vi "Close_loop_Position_Control_of_Tip.vi"() -> ()   [LabVIEW 2019]
uses:
  <vilib>/FPGAPlugInAG/sbRIO-9629/niLvFpga_Open_sbRIO-9629.vi
  <vilib>/rvi/interface/common/dynamic/niFpgaDynamicAddResources.vi
  <vilib>/imath/engines/lvmath2/RunTimeEngine/Managers/WorkSpace/UID Generator.vi
  <vilib>/imath/engines/lvmath2/RunTimeEngine/IndexRead/NIMS V(S).vi
  <instcachedir>/0/NIMS V(S)_0488751826AF41519A22953C041130DC.lvgen/NIMS V(S)_0488751826AF41519A22953C041130DC_000.vi
  <vilib>/imath/engines/lvmath2/RunTimeEngine/BuiltInFunctions/atan2/NIMS_atan2.vi
  <instcachedir>/0/NIMS_atan2_A91AA4A7D42247EDBE8F76DB99AF04A4.lvgen/NIMS_atan2_A91AA4A7D42247EDBE8F76DB99AF04A4_000.vi
  <vilib>/imath/engines/lvmath2/RunTimeEngine/RunTimeType/NIMS_RunTimeType_From StrictType (excl LVString).vi
  <instcachedir>/0/NIMS_RunTimeType_From StrictType (excl LVString)_D8AFBA86A94845AAA577C895450664BD.lvgen/NIMS_RunTimeType_From StrictType (excl LVString)_D8AFBA86A94845AAA577C895450664BD_000.vi
  <vilib>/imath/engines/lvmath2/RunTimeEngine/ErrorHandling/NIMS_Create Error From Enums.vi
  <vilib>/imath/engines/lvmath2/RunTimeEngine/LocalVariableDefStatement/MC_LocalVariableDefStatement_Display.vi
  <vilib>/imath/engines/lvmath2/RunTimeEngine/BuiltInFunctions/atan/NIMS_atan(C).vi
  <instcachedir>/0/NIMS_atan(C)_0A85D365582D4E8AB3874BC9125E138E.lvgen/NIMS_atan(C)_0A85D365582D4E8AB3874BC9125E138E_001.vi
  <vilib>/imath/engines/lvmath2/RunTimeEngine/BuiltInFunctions/cross/NIMS_cross(GV,GV).vi
  <instcachedir>/0/NIMS_cross(GV,GV)_6F1F1C643EFF41C8A983D972A94A5A15.lvgen/NIMS_cross(GV,GV)_6F1F1C643EFF41C8A983D972A94A5A15_000.vi
  <vilib>/imath/engines/lvmath2/RunTimeEngine/BuiltInFunctions/norm/NIMS_norm(GV,DBL).vi
  <instcachedir>/0/NIMS_norm(GV,DBL)_4A8B6F23BC0A47549B8AB805006257D9.lvgen/NIMS_norm(GV,DBL)_4A8B6F23BC0A47549B8AB805006257D9_000.vi
  <vilib>/imath/engines/lvmath2/RunTimeEngine/ArithmeticOperatorToken/NIMS_ArithmeticOperator_multmx-internal.vi
  <instcachedir>/0/NIMS_ArithmeticOperator_multmx-internal_9E91BA3A2DCB4083AAD724A04442A6F7.lvgen/NIMS_ArithmeticOperator_multmx-internal_9E91BA3A2DCB4083AAD724A04442A6F7_004.vi
  <vilib>/imath/engines/lvmath2/RunTimeEngine/BuiltInFunctions/cos/NIMS_cos(C).vi
  <instcachedir>/0/NIMS_cos(C)_BED070B05FDB4939A63CB05E18805866.lvgen/NIMS_cos(C)_BED070B05FDB4939A63CB05E18805866_001.vi
  <vilib>/imath/engines/lvmath2/RunTimeEngine/BuiltInFunctions/sin/NIMS_sin(C).vi
  <instcachedir>/0/NIMS_sin(C)_6504C6AC704B4661870B0E93397B11C4.lvgen/NIMS_sin(C)_6504C6AC704B4661870B0E93397B11C4_001.vi
  <vilib>/imathl/engines/lvmath/Functions/Error Handling/Create Error.vi
  <vilib>/imath/engines/lvmath2/RunTimeEngine/ArithmeticOperatorToken/NIMS_ArithmeticOperator_multmx(M,CV)-internal.vi
  <instcachedir>/0/NIMS_ArithmeticOperator_multmx(M,CV)-internal_2C55777844884EEDB828A940D397C7D0.lvgen/NIMS_ArithmeticOperator_multmx(M,CV)-internal_2C55777844884EEDB828A940D397C7D0_002.vi
  <instcachedir>/0/NIMS_norm(GV,DBL)_4A8B6F23BC0A47549B8AB805006257D9.lvgen/NIMS_norm(GV,DBL)_4A8B6F23BC0A47549B8AB805006257D9_001.vi
  <vilib>/imath/engines/lvmath2/RunTimeEngine/Managers/SymbolTable/Clear UID.vi
  <vilib>/imath/engines/lvmath2/RunTimeEngine/NodeEndStatement/NIMS_NodeEndStatement_Output.vi
  <instcachedir>/0/NIMS_NodeEndStatement_Output_53EC0D466D134D7ABD903AC30B43404B.lvgen/NIMS_NodeEndStatement_Output_53EC0D466D134D7ABD903AC30B43404B_001.vi
  <vilib>/imath/engines/lvmath2/RunTimeEngine/ErrorHandling/NIMS_Finalize Error.vi
  <vilib>/Utility/error.llb/Error Cluster From Error Code.vi
  <vilib>/rvi/errors/niLvFpgaAdjustHostInterfaceError.vi
  <vilib>/FPGAPlugInAG/Dynamic/niLvFpga_Close_Dynamic.vi
  <vilib>/rvi/interface/nirviOpenFPGA/nirviOpenFPGA.xnode
  FPGA Bitfiles/fcmsinglesection_FPGATarget_CloseLoopMotorTu_eGt+d+EV+VE.lvbitx
  Close_Loop_Motor_Tune.vi
  <vilib>/rvi/interface/nirviReadWriteControl/nirviReadWriteControl.xnode
  <vilib>/rvi/interface/nirviCloseFPGA/nirviCloseFPGA.xnode
  NiFpgaLv.dll
  <vilib>/rvi/interface/Simulation/niFpgaSimulationCallBeginRW.vi
  <vilib>/imath/engines/lvmath2/RunTimeEngine/Managers/SymbolTable/NIMS_WorkSpace.lvlib
panel:
  in  "Kp":dbl[](array[numeric])
  in  "Motor3_KP":sgl
  in  "Motor2_KP":sgl
  in  "Motor1_KP":sgl
  in  "Position Reset 2_e":bool
  out "Theta 3 (error)":dbl
  out "Theta 2 (error)":dbl
  out "Theta 1 (error)":dbl
  out "alpha (error)":dbl
  out "L_v (error)":dbl
  out "Error Indicator":bool
  out "Error":dbl[](array[numeric])
  out "error out 2":errorcluster
  out "Y Position(mm) marker 25":dbl
  out "X Position(mm) marker 25":dbl
  out "Z Position(mm) marker 25":dbl
  out "Actual Tip Coordinates(m)":dbl[](array[numeric])
  out "LED ID 2":i32
  out "FRAME 2":string
  out "data out 2":string
  in  "Desired Tip position (m)":dbl[](array[numeric])
  out "L1 (m)":dbl
  out "L2 (m)":dbl
  out "L3 (m)":dbl
  out "Theta 1":dbl
  out "Theta 2":dbl
  out "Theta 3":dbl
  in  "Position Reset":bool
  out "output variable":dbl
  out "output variable 2":dbl
  out "output variable 3":dbl
  out "alpha":dbl
  out "L_v":dbl
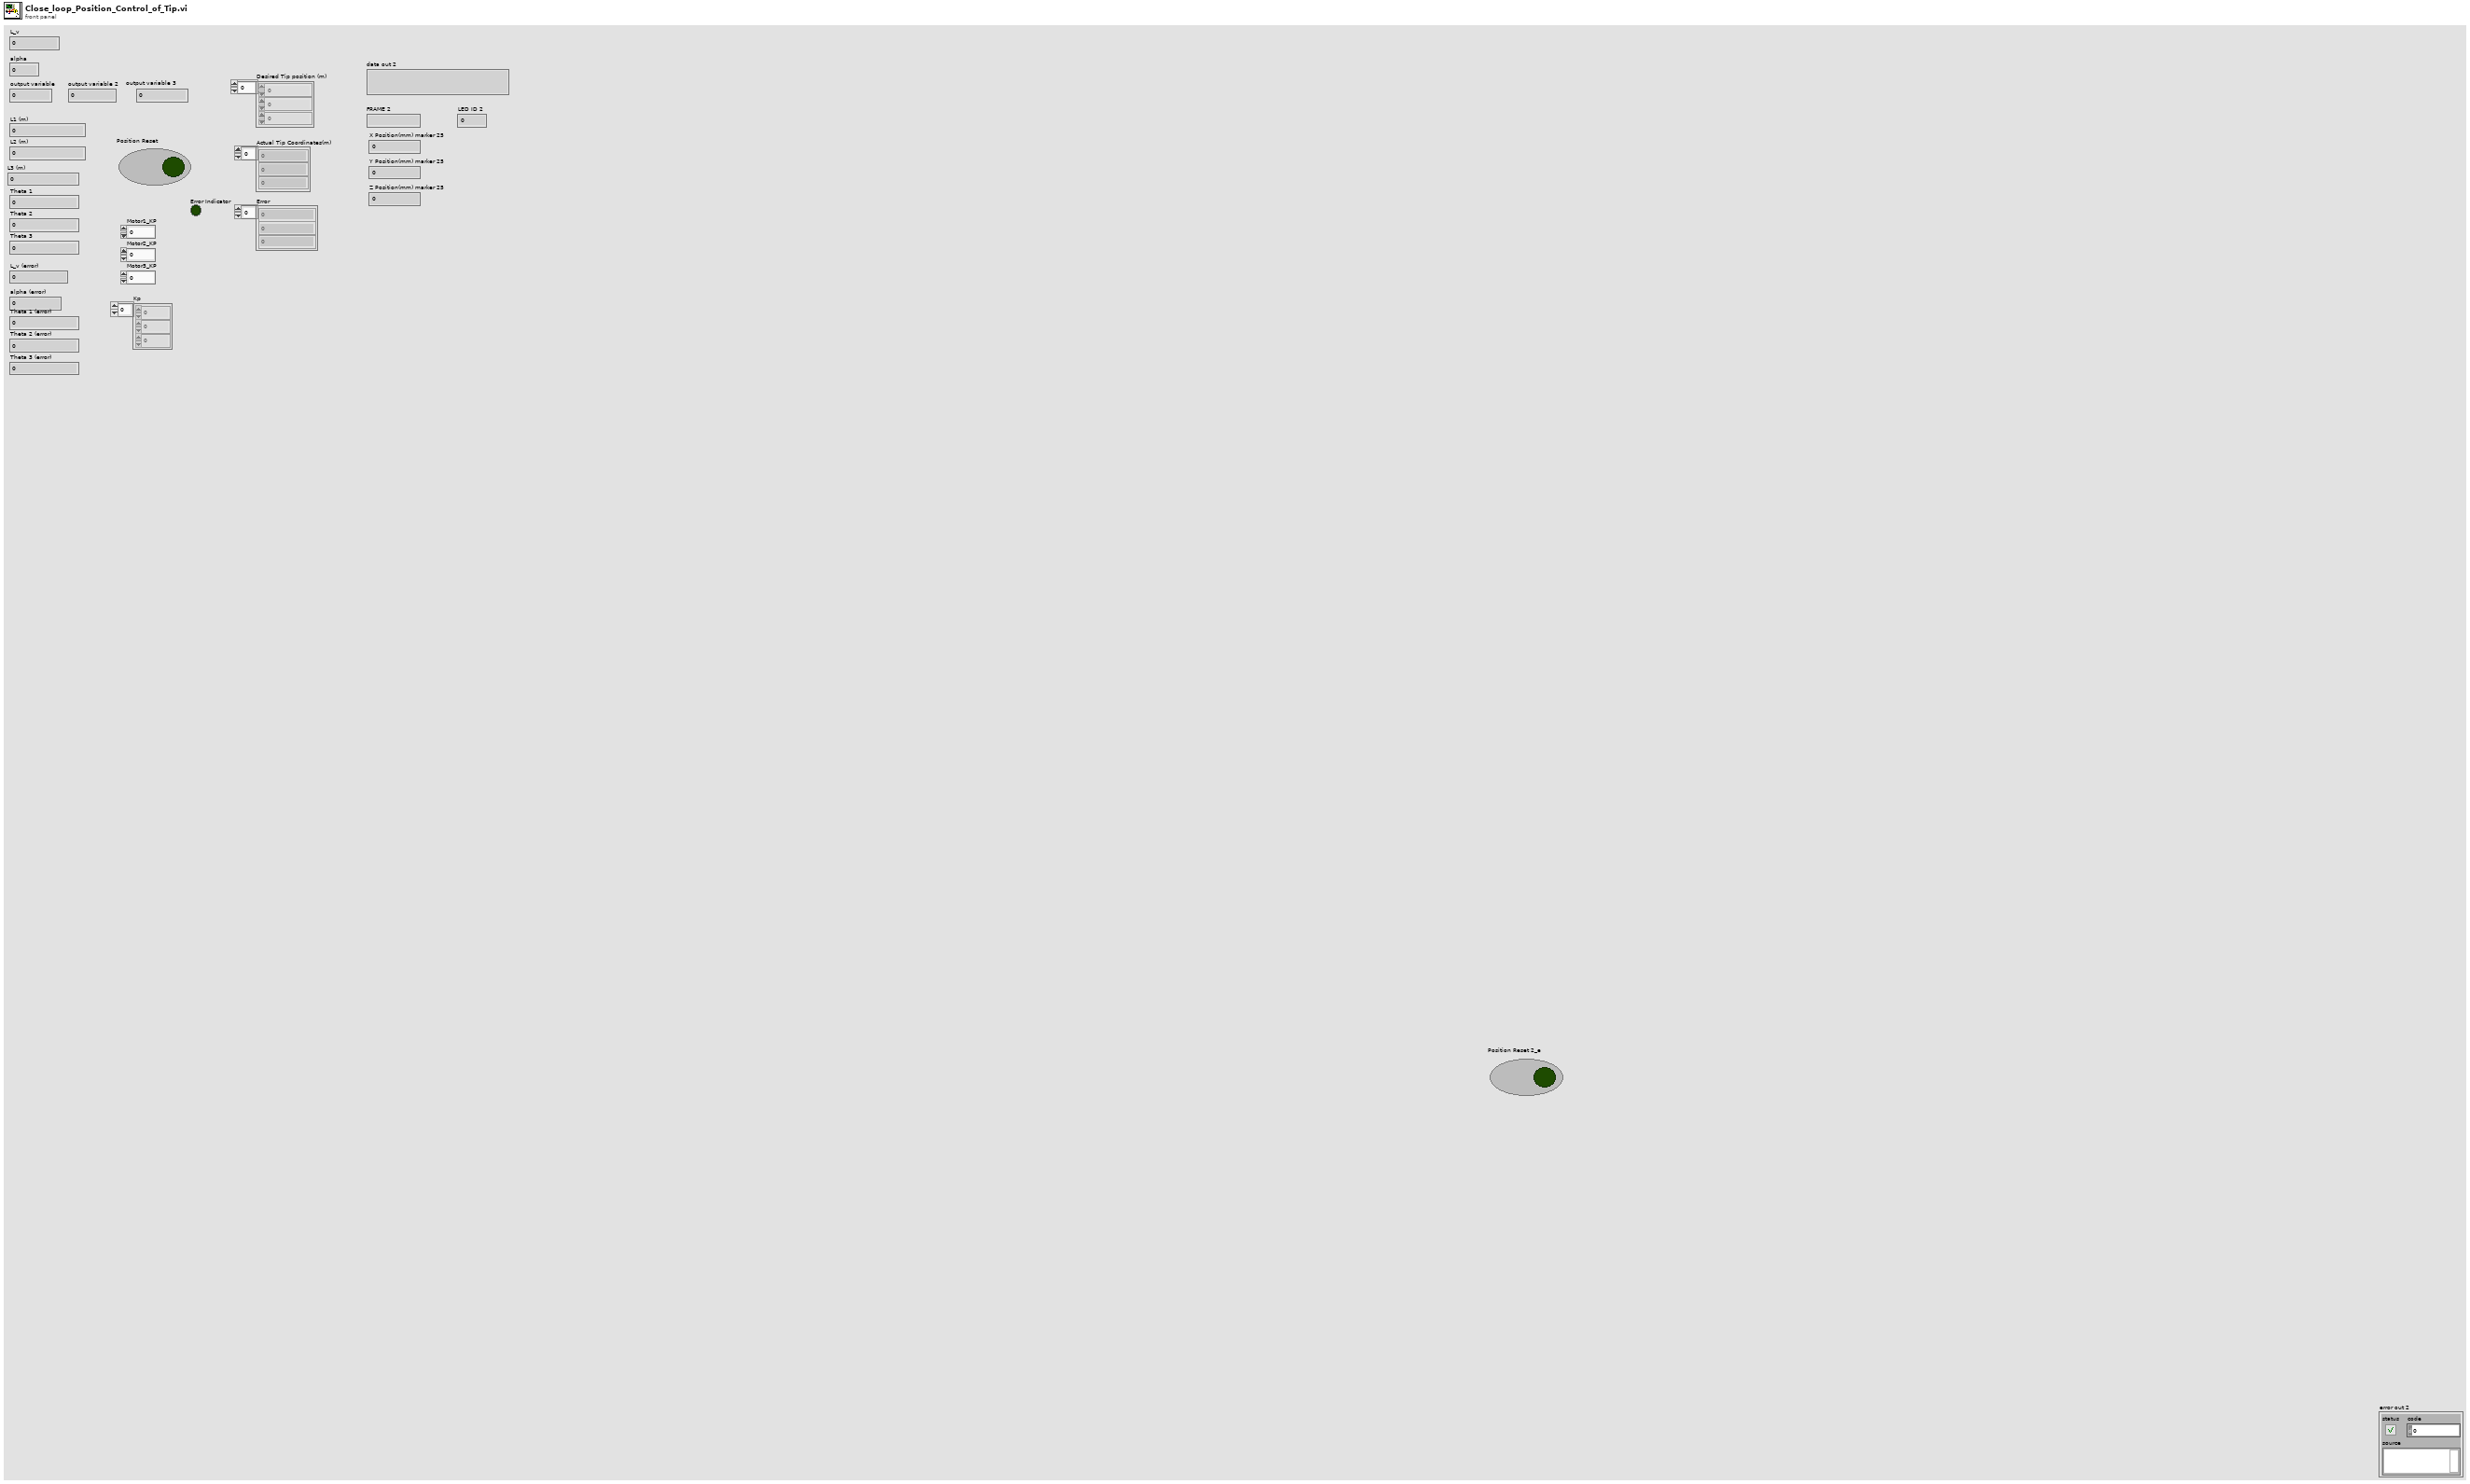
[diagram p1: front panel]
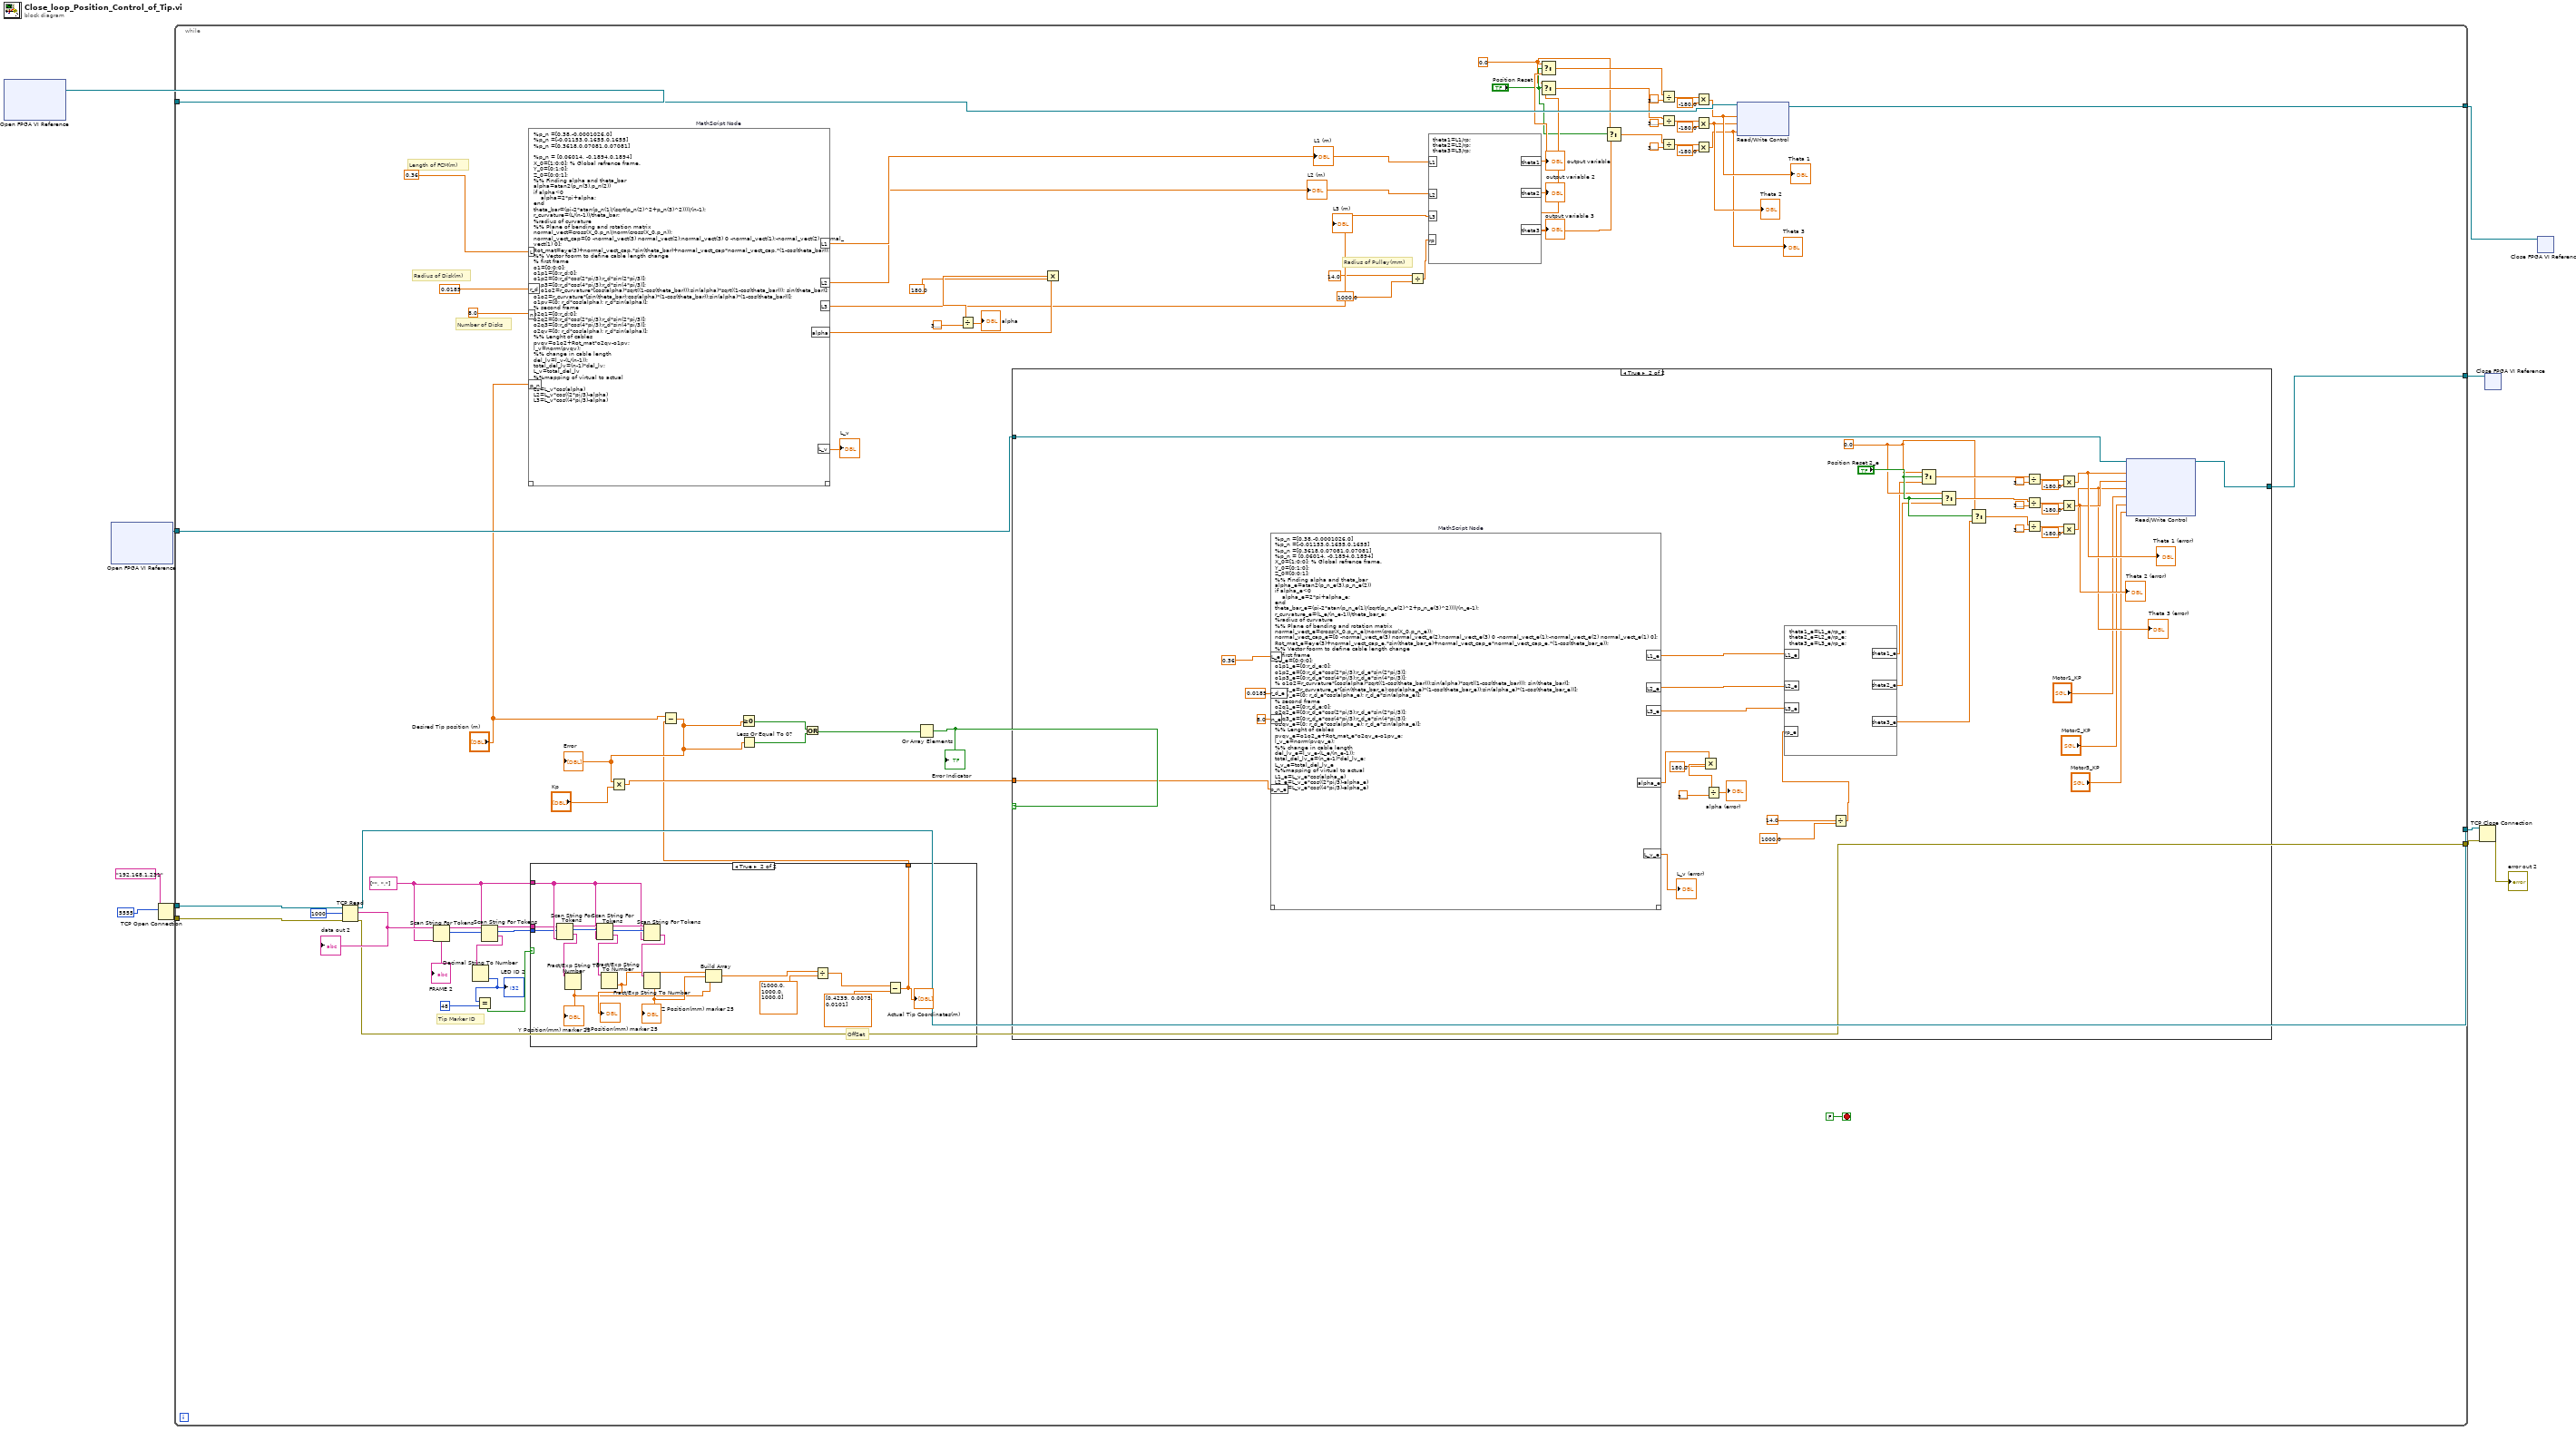
[diagram p0: block diagram]
diagram:
  n1 = xnode "Open FPGA VI Reference"() -> ("FPGA VI Reference Out"=w3:refnum<k20>)  [unwired: 2 in, 1 out]
  n2 = xnode "Open FPGA VI Reference"() -> ("FPGA VI Reference Out"=w1:refnum<k20>)  [unwired: 2 in, 1 out]
  n3 = TCP Open Connection(address="192.168.1.231", remote port or service name=u16 5555) -> (connection ID=w7:refnum<k5>, error out=w8:errorcluster)  [unwired: 3 in]
  n4 = while {
    tunnel: w3 -> [w73]
    tunnel: [w72] -> w11
    tunnel: w8 -> [w33]
    tunnel: w7 -> [w32]
    tunnel: [w31] -> w5
    tunnel: [w30] -> w4
    tunnel: [w22] -> w2
    tunnel: w1 -> [w21]
    stop <- FALSE stop-if-true
    w14 = string[] ["", ","] ("delimiters (\\s,\\t,\\r,\\n)")
    w55 = 0.0 ("t")
    # "Tip Marker ID"
    # "Length of FCM(m)"
    # "Radius of Disk(m)"
    # "Number of Disks"
    # "Radius of Pulley(mm)"
    n5 = TCP Read(connection ID=w32, bytes to read=1000, error in (no error)=w33) -> (connection ID out=w31:refnum<k5>, data out=w40:string, error out=w30:errorcluster)  [unwired: 2 in]
    "data out 2" <- w40
    n6 = Scan String For Tokens(6:w14, 9:w40) -> (1:→"FRAME 2":string, 2:w38:i32, 3:w37:string)  [unwired: 4 in, 1 out]
    n7 = Scan String For Tokens(6:w14, 8:w38, 9:w37) -> (1:w36:string, 2:w15:i32, 3:w16:string)  [unwired: 3 in, 1 out]
    n8 = Decimal String To Number(string=w36) -> (number=w17:i32)  [unwired: 2 in, 1 out]
    "LED ID 2" <- w17
    n9 = Equal?(x=w17, y=48) -> (x = y?=w34:bool)
    n10 = mathscript code="%p_n =[0.38,-0.0001026,0] \n%p_n =[-0.01153,0.1655,0.1655] \n%p_n =[0.3618,0.07081,0.07081] \n\n%p_n = [0.06014, -0.1894,0.1894]\nX_0=[1;0;0]; % Global refrence frame.\nY_0=[0;1;0];\nZ_0=[0;0;1];\n%% Finding alpha and theta_bar\nalpha=atan2(p_n(3),p_n(2))\nif alpha<0\n    alpha=2*pi+alpha;\nend\ntheta_bar=(pi-2*atan(p_n(1)/(sqrt(p_n(2)^2+p_n(3)^2))))/(n-1);\nr_curvature=(L/(n-1))/theta_bar; \n%radius of curvature\n%% Plane of bending and rotation matrix\nnormal_vect=cross(X_0,p_n)/norm(cross(X_0,p_n));\nnormal_vect_cap=[0 -normal_vect(3) normal_vect(2);normal_vect(3) 0 -normal_vect(1);-normal_vect(2) normal_vect(1) 0];\nRot_mat=eye(3)+normal_vect_cap.*sin(theta_bar)+normal_vect_cap*normal_vect_cap.*(1-cos(theta_bar));\n%% Vector foorm to define cable length change\n% first frame\no1=[0;0;0];\no1p1=[0;r_d;0];\no1p2=[0;r_d*cos(2*pi/3);r_d*sin(2*pi/3)];\no1p3=[0;r_d*cos(4*pi/3);r_d*sin(4*pi/3)];\n% o1o2=r_curvature*[cos(alpha)*sqrt((1-cos(theta_bar)));sin(alpha)*sqrt((1-cos(theta_bar))); sin(theta_bar)];\no1o2=r_curvature*[sin(theta_bar);cos(alpha)*(1-cos(theta_bar));sin(alpha)*(1-cos(theta_bar))];\no1pv=[0; r_d*cos(alpha); r_d*sin(alpha)];\n% second frame\no2q1=[0;r_d;0];\no2q2=[0;r_d*cos(2*pi/3);r_d*sin(2*pi/3)];\no2q3=[0;r_d*cos(4*pi/3);r_d*sin(4*pi/3)];\no2qv=[0; r_d*cos(alpha); r_d*sin(alpha)];\n%% Lenght of cables\npvqv=o1o2+Rot_mat*o2qv-o1pv;\nl_v=norm(pvqv);\n%% change in cable length\ndel_lv=l_v-(L/(n-1));\ntotal_del_lv=(n-1)*del_lv;\nL_v=total_del_lv\n%%mapping of virtual to actual\n\nL1=L_v*cos(alpha)\nL2=L_v*cos((2*pi/3)-alpha)\nL3=L_v*cos((4*pi/3)-alpha)"("L"=0.36 ("Length of the FCM (mm)"), "r_d"=0.0185, "n"=8.0 ("Number of Disks"), "p_n"="Desired Tip position (m)") -> ("L_v"=→"L_v":dbl, "alpha"=w48:dbl, "L1"=w45:dbl, "L2"=w44:dbl, "L3"=w43:dbl)  [unwired: 1 in, 1 out]
    "L1 (m)" <- w45
    "L2 (m)" <- w44
    "L3 (m)" <- w43
    n11 = case shown="True" w34 {
      tunnel: w16 -> [_ w698]
      tunnel: w15 -> [_ w697]
      tunnel: w14 -> [_ w699]
      tunnel: [_ w692] -> w12
      frame False {
      }
      frame True {
        # "OffSet"
        n12 = Scan String For Tokens(6:w699, 8:w697, 9:w698) -> (1:w702:string, 2:w705:i32, 3:w707:string)  [unwired: 3 in, 1 out]
        n13 = Fract/Exp String To Number(string=w702) -> (number=w690:dbl)  [unwired: 3 in, 1 out]
        "Y Position(mm) marker 25" <- w690
        n14 = Scan String For Tokens(6:w699, 8:w705, 9:w707) -> (1:w703:string, 2:w704:i32, 3:w706:string)  [unwired: 3 in, 1 out]
        n15 = Fract/Exp String To Number(string=w703) -> (number=w700:dbl)  [unwired: 3 in, 1 out]
        "X Position(mm) marker 25" <- w700
        n16 = Scan String For Tokens(6:w699, 8:w704, 9:w706) -> (1:w701:string)  [unwired: 3 in, 3 out]
        n17 = Fract/Exp String To Number(string=w701) -> (number=w691:dbl)  [unwired: 3 in, 1 out]
        "Z Position(mm) marker 25" <- w691
        n18 = Build Array(w700, w691, w690) -> (w696:dbl[])
        n19 = Divide(x=w696, y=dbl[] [1000.0, 1000.0, 1000.0]) -> (x/y=w694:dbl[])
        n20 = Subtract(x=w694, y=dbl[] [0.4239, 0.0075, 0.0101]) -> (x-y=w692:dbl[])
        "Actual Tip Coordinates(m)" <- w692
      }
    }
    n21 = Subtract(x="Desired Tip position (m)", y=w12) -> (x-y=w19:dbl[])
    "Error" <- w19
    n22 = Multiply(x=w19, y="Kp") -> (x*y=w18:dbl[])
    n23 = Greater Or Equal To 0?(x=w19) -> (x >= 0?=w29:bool[])
    n24 = Less Or Equal To 0?(x=w19) -> (x <= 0?=w28:bool[])
    n25 = Or(x=w29, y=w28) -> (x .or. y?=w27:bool[])
    n26 = Or Array Elements(Boolean array=w27) -> (logical OR=w26:bool)
    "Error Indicator" <- w26
    n27 = case shown="True" w26 {
      tunnel: w18 -> [_ w118]
      tunnel: [w77 w85] -> w22
      tunnel: w21 -> [w77 w84]
      frame False {
      }
      frame True {
        w92 = 0.0 ("t")
        n28 = mathscript code="%p_n =[0.38,-0.0001026,0] \n%p_n =[-0.01153,0.1655,0.1655] \n%p_n =[0.3618,0.07081,0.07081] \n%p_n = [0.06014, -0.1894,0.1894]\nX_0=[1;0;0]; % Global refrence frame.\nY_0=[0;1;0];\nZ_0=[0;0;1];\n%% Finding alpha and theta_bar\nalpha_e=atan2(p_n_e(3),p_n_e(2))\nif alpha_e<0\n    alpha_e=2*pi+alpha_e;\nend\ntheta_bar_e=(pi-2*atan(p_n_e(1)/(sqrt(p_n_e(2)^2+p_n_e(3)^2))))/(n_e-1);\nr_curvature_e=(L_e/(n_e-1))/theta_bar_e; \n%radius of curvature\n%% Plane of bending and rotation matrix\nnormal_vect_e=cross(X_0,p_n_e)/norm(cross(X_0,p_n_e));\nnormal_vect_cap_e=[0 -normal_vect_e(3) normal_vect_e(2);normal_vect_e(3) 0 -normal_vect_e(1);-normal_vect_e(2) normal_vect_e(1) 0];\nRot_mat_e=eye(3)+normal_vect_cap_e.*sin(theta_bar_e)+normal_vect_cap_e*normal_vect_cap_e.*(1-cos(theta_bar_e));\n%% Vector foorm to define cable length change\n% first frame\no1_e=[0;0;0];\no1p1_e=[0;r_d_e;0];\no1p2_e=[0;r_d_e*cos(2*pi/3);r_d_e*sin(2*pi/3)];\no1p3_e=[0;r_d_e*cos(4*pi/3);r_d_e*sin(4*pi/3)];\n% o1o2=r_curvature*[cos(alpha)*sqrt((1-cos(theta_bar)));sin(alpha)*sqrt((1-cos(theta_bar))); sin(theta_bar)];\no1o2_e=r_curvature_e*[sin(theta_bar_e);cos(alpha_e)*(1-cos(theta_bar_e));sin(alpha_e)*(1-cos(theta_bar_e))];\no1pv_e=[0; r_d_e*cos(alpha_e); r_d_e*sin(alpha_e)];\n% second frame\no2q1_e=[0;r_d_e;0];\no2q2_e=[0;r_d_e*cos(2*pi/3);r_d_e*sin(2*pi/3)];\no2q3_e=[0;r_d_e*cos(4*pi/3);r_d_e*sin(4*pi/3)];\no2qv_e=[0; r_d_e*cos(alpha_e); r_d_e*sin(alpha_e)];\n%% Lenght of cables\npvqv_e=o1o2_e+Rot_mat_e*o2qv_e-o1pv_e;\nl_v_e=norm(pvqv_e);\n%% change in cable length\ndel_lv_e=l_v_e-(L_e/(n_e-1));\ntotal_del_lv_e=(n_e-1)*del_lv_e;\nL_v_e=total_del_lv_e\n%%mapping of virtual to actual\nL1_e=L_v_e*cos(alpha_e)\nL2_e=L_v_e*cos((2*pi/3)-alpha_e)\nL3_e=L_v_e*cos((4*pi/3)-alpha_e)"("L_e"=0.36 ("L"), "r_d_e"=0.0185 ("r_d"), "n_e"=8.0 ("n"), "p_n_e"=w118) -> ("L_v_e"=→"L_v (error)":dbl, "alpha_e"=w113:dbl, "L1_e"=w111:dbl, "L2_e"=w110:dbl, "L3_e"=w109:dbl)  [unwired: 1 in, 1 out]
        n29 = Multiply(x=w113, y=180.0) -> (x*y=w115:dbl)
        n30 = Divide(x=w115, y=3.141592653589793) -> (x/y=→"alpha (error)":dbl)
        n31 = Divide(x=14.0 ("Radius of pulley (mm)"), y=1000.0) -> (x/y=w107:dbl)
        n32 = formula code="theta1_e=L1_e/rp_e;\ntheta2_e=L2_e/rp_e;\ntheta3_e=L3_e/rp_e;"("L1_e"=w111, "L2_e"=w110, "L3_e"=w109, "rp_e"=w107) -> ("theta1_e"=w88:dbl, "theta2_e"=w87:dbl, "theta3_e"=w86:dbl)
        n33 = Select(t=w92, s="Position Reset 2_e", f=w88) -> (s? t:f=w96:dbl)
        n34 = Select(t=w92, s="Position Reset 2_e", f=w87) -> (s? t:f=w95:dbl)
        n35 = Select(t=w92, s="Position Reset 2_e", f=w86) -> (s? t:f=w94:dbl)
        n36 = Divide(x=w96, y=3.141592653589793) -> (x/y=w104:dbl)
        n37 = Divide(x=w95, y=3.141592653589793) -> (x/y=w101:dbl)
        n38 = Divide(x=w94, y=3.141592653589793) -> (x/y=w98:dbl)
        n39 = Multiply(x=w104, y=-180.0) -> (x*y=w91:dbl)
        "Theta 1 (error)" <- w91
        n40 = Multiply(x=w101, y=-180.0) -> (x*y=w90:dbl)
        "Theta 2 (error)" <- w90
        n41 = Multiply(x=w98, y=-180.0) -> (x*y=w89:dbl)
        "Theta 3 (error)" <- w89
        n42 = xnode "Read/Write Control"("FPGA VI Reference In"=w84, "desired angle (error)"=w91, "desired angle 2(error)"=w90, "desired angle 3(error)"=w89, "Motor1_KP"="Motor1_KP", "Motor2_KP"="Motor2_KP", "Motor3_KP"="Motor3_KP") -> ("FPGA VI Reference Out"=w85:refnum<k20>)  [unwired: 1 in, 1 out]
      }
    }
    n43 = Multiply(x=w48, y=180.0) -> (x*y=w50:dbl)
    n44 = Divide(x=w50, y=3.141592653589793) -> (x/y=→"alpha":dbl)
    n45 = Divide(x=14.0, y=1000.0) -> (x/y=w75:dbl)
    n46 = formula code="theta1=L1/rp;\ntheta2=L2/rp;\ntheta3=L3/rp;"("L1"=w45, "L2"=w44, "L3"=w43, "rp"=w75) -> ("theta1"=w62:dbl, "theta2"=w59:dbl, "theta3"=w57:dbl)
    "output variable" <- w62
    "output variable 2" <- w59
    "output variable 3" <- w57
    n47 = Select(t=w55, s="Position Reset", f=w62) -> (s? t:f=w61:dbl)
    n48 = Select(t=w55, s="Position Reset", f=w59) -> (s? t:f=w60:dbl)
    n49 = Select(t=w55, s="Position Reset", f=w57) -> (s? t:f=w58:dbl)
    n50 = Divide(x=w61, y=3.141592653589793) -> (x/y=w70:dbl)
    n51 = Divide(x=w60, y=3.141592653589793) -> (x/y=w67:dbl)
    n52 = Divide(x=w58, y=3.141592653589793) -> (x/y=w64:dbl)
    n53 = Multiply(x=w70, y=-180.0) -> (x*y=w54:dbl)
    "Theta 1" <- w54
    n54 = Multiply(x=w67, y=-180.0) -> (x*y=w53:dbl)
    "Theta 2" <- w53
    n55 = Multiply(x=w64, y=-180.0) -> (x*y=w52:dbl)
    "Theta 3" <- w52
    n56 = xnode "Read/Write Control"("FPGA VI Reference In"=w73, "desired angle"=w54, "desired angle 2"=w53, "desired angle 3"=w52) -> ("FPGA VI Reference Out"=w72:refnum<k20>)  [unwired: 1 in, 1 out]
  }
  n57 = TCP Close Connection(connection ID=w5, error in (no error)=w4) -> (error out=→"error out 2":errorcluster)  [unwired: 1 in, 1 out]
  n58 = xnode "Close FPGA VI Reference"("FPGA VI Reference In"=w2) -> ()  [unwired: 1 in, 1 out]
  n59 = xnode "Close FPGA VI Reference"("FPGA VI Reference In"=w11) -> ()  [unwired: 1 in, 1 out]
